vi "BT Example 6 - Parallel.vi"() -> ()   [LabVIEW 2021]
uses:
  Support/Nodes/abs_Node/Status.ctl
  Blackboard/Blackboard.lvclass
  Support/Nodes/Decorators/Repeater/Support/Finish On - Type.ctl
  Support/Nodes/Composites/abs_Parallel/Support/Status Calculation.ctl
  System/bt_System.lvclass
  Blackboard/Blackboard.lvclass/Blackboard.ctl
  Support/Nodes/Leaves/abs_Type Leaf/abs_Type Leaf.lvclass/abs_Type Leaf.ctl
  Blackboard/Get Value Type/Get I32.vi
  <vilib>/TSA/Abstract Data Classes/Abs_Types/I32 Integer/Static Read.vi
  Blackboard/Support/Index Group.vi
  Blackboard/Support/Index Tags.vi
  Support/Nodes/Leaves/abs_Type Leaf/Properties/Write Value Class.vi
  <vilib>/TSA/Omni-Bus/Local Bus/Support/I32/Local Bus_I32.lvclass
  C:/Program Files (x86)/National Instruments/LabVIEW 2021/vi.lib/TSA/Abstract Data Classes/Abs_Types/Value/Abs_Value.lvclass
  <vilib>/TSA/Abstract Data Classes/Abs_Types/I32 Integer/Abs_I32 Integer.lvclass
  Support/Nodes/Leaves/Test Boolean/Test Abs_Boolean.lvclass
  C:/Users/Tim/Documents/GitHub/LV_Behaviour_Tree/Source/Support/Nodes/abs_Node/bt_Node.lvclass
  C:/Users/Tim/Documents/GitHub/LV_Behaviour_Tree/Source/Support/Nodes/Leaves/abs_Type Leaf/abs_Type Leaf.lvclass
  <vilib>/TSA/Abstract Data Classes/Abs_Types/Boolean/Abs_Boolean.lvclass
  C:/Program Files (x86)/National Instruments/LabVIEW 2021/vi.lib/TSA/Abstract Data Classes/Abs_Types/Type/Abs_Type.lvclass
  <vilib>/TSA/Omni-Bus/Local Bus/Support/Initialise DVR's.vi
  <vilib>/TSA/Abstract Data Classes/Functions/Math/Support/Increment/I32/Method.vi
  <vilib>/TSA/Abstract Data Classes/Constants/Support/I32/I32.vi
  <vilib>/TSA/Abstract Data Classes/Functions/Math/Support/Add/I32/Method_Const.vi
  <vilib>/TSA/Abstract Data Classes/Functions/Compare/Support/Less/I32/Method_Const.vi
  <vilib>/TSA/Abstract Data Classes/Abs_Types/Value/Abs_Value.lvclass
  <vilib>/TSA/Abstract Data Classes/Abs_Types/Type/Abs_Type.lvclass
  <vilib>/TSA/Omni-Bus/Local Bus/Support/DBL/Local Bus_DBL.lvclass
  <vilib>/TSA/Omni-Bus/Local Bus/Support/SGL/Local Bus_SGL.lvclass
  <vilib>/TSA/Omni-Bus/Local Bus/Support/EXT/Local Bus_EXT.lvclass
  <vilib>/TSA/Omni-Bus/Local Bus/Support/Bool/Local Bus_Boolean.lvclass
  <vilib>/TSA/Omni-Bus/Local Bus/Support/STR/Local Bus_String.lvclass
  <vilib>/TSA/Omni-Bus/Local Bus/Support/Variant/Local Bus_Variant.lvclass
  <vilib>/TSA/Omni-Bus/Local Bus/Support/WFM/Local Bus_Waveform.lvclass
  <vilib>/TSA/Omni-Bus/Local Bus/Support/Time/Local Bus_Time.lvclass
  <vilib>/TSA/Omni-Bus/Local Bus/Support/U8/Local Bus_U8.lvclass
  <vilib>/TSA/Omni-Bus/Local Bus/Support/U16/Local Bus_U16.lvclass
  <vilib>/TSA/Omni-Bus/Local Bus/Support/U32/Local Bus_U32.lvclass
  <vilib>/TSA/Omni-Bus/Local Bus/Support/U64/Local Bus_U64.lvclass
  <vilib>/TSA/Omni-Bus/Local Bus/Support/I8/Local Bus_I8.lvclass
  <vilib>/TSA/Omni-Bus/Local Bus/Support/I16/Local Bus_I16.lvclass
  <vilib>/TSA/Omni-Bus/Local Bus/Support/I64/Local Bus_I64.lvclass
  <vilib>/TSA/Omni-Bus/Local Bus/Support/CSGL/Local Bus_CSGL.lvclass
  <vilib>/TSA/Omni-Bus/Local Bus/Support/CDBL/Local Bus_CDBL.lvclass
  <vilib>/TSA/Omni-Bus/Local Bus/Support/CEXT/Local Bus_CEXT.lvclass
  BT.lvlib
  Support/Nodes/Decorators/Repeater/bt_Repeater.lvclass
  Support/Nodes/Composites/abs_Parallel/bt_Parallel.lvclass
  <vilib>/TSA/Abstract Data Classes/Functions/Math/Support/Increment/I32/Increment_I32.lvclass
  <vilib>/TSA/Abstract Data Classes/Functions/Compare/Support/Less/I32/Less_I32.lvclass
  Support/Nodes/abs_Node/bt_Node.lvclass
  <vilib>/TSA/Abstract Data Classes/Constants/Support/I32/Const_I32.lvclass
  <vilib>/TSA/Abstract Data Classes/Functions/Math/Support/Add/I32/Add_I32.lvclass
panel:
  out "Status":T1
  out "Counts":i32[](array[numeric])
  in  "stop":bool
  # "Count 1"
  # "Count 2"
  # "Finish Count"
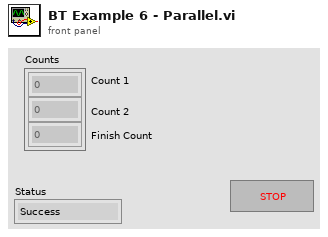
[diagram p1: front panel]
types:
  T1 = typedef "BT.lvlib/bt_Node.lvclass/Status.ctl" = enum16{"Success", "Failure", "Running"}
  T2 = typedef "BT.lvlib/bt_Parallel.lvclass/Status Calculation.ctl" = enum16{"Succeed on All Succeed", "Failure on All Failure", "Succeed on Any Succeed", "Failure on Any Failure"}
  T3 = typedef "BT.lvlib/bt_Repeater.lvclass/Finish On - Type.ctl" = enum16{"Success", "Failure", "Never"}
  T4 = typedef "Add_I32.lvclass/Abs_Type.ctl" = refnum<class "Abs_I32 Integer.lvclass">
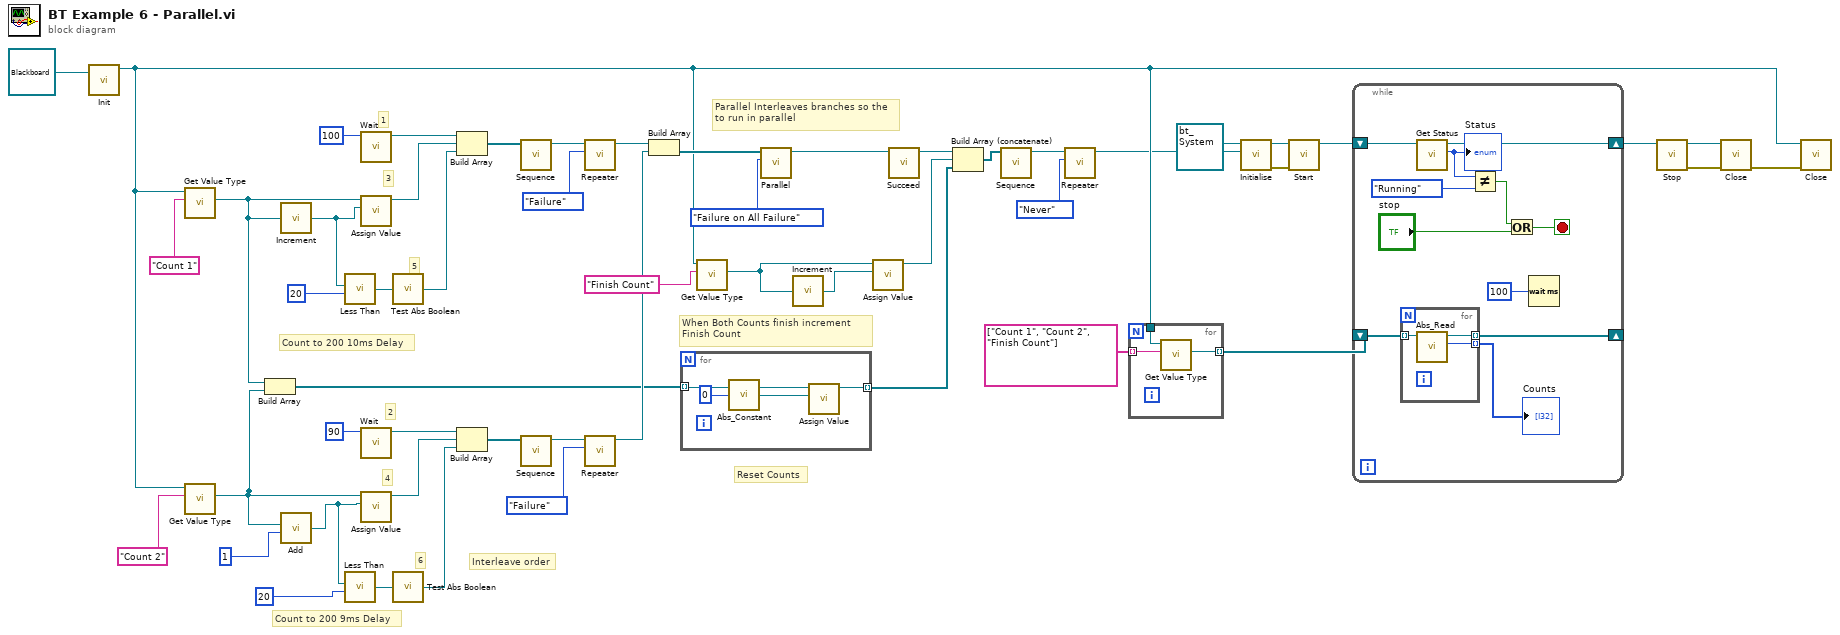
[diagram p0: block diagram]
diagram:
  # "Interleave order"
  # "6"
  # "5"
  # "4"
  # "3"
  # "2"
  # "1"
  # "Count to 200 9ms Delay"
  # "Parallel Interleaves branches so the\nto run in parallel"
  # "Reset Counts"
  # "When Both Counts finish increment\nFinish Count"
  # "Count to 200 10ms Delay"
  n1 = call-dynamic "Init.vi"("bt_Blackboard in"=refnum<class "Blackboard.lvclass"> refnum) -> ("bt_Blackboard out"=w20:refnum<class "Blackboard.lvclass">)  [unwired: 9 in, 1 out]
  n2 = call-poly "Get Value Type.vi"("Tag"="Count 1", "Blackboard in"=w20) -> ("Value"=w13:refnum<class "Abs_I32 Integer.lvclass">)  [unwired: 6 in, 3 out]
  n3 = call-poly "Get Value Type.vi"("Tag"="Count 2", "Blackboard in"=w20) -> ("Value"=w12:refnum<class "Abs_I32 Integer.lvclass">)  [unwired: 6 in, 3 out]
  n4 = Build Array(w13, w12) -> (w11:refnum<class "Abs_I32 Integer.lvclass">[])
  n5 = call-poly <vilib>:"Increment.vi"("Value"=w13) -> ("Result"=w28:refnum<class "Abs_I32 Integer.lvclass">)  [unwired: 4 in]
  n6 = call-poly <vilib>:"Add.vi"("Value"=1, "Input A"=w12) -> ("Result"=w31:T4)  [unwired: 4 in]
  n7 = call-poly <vilib>:"Less Than.vi"("Value"=20, "Value A"=w28) -> ("Result"=w29:refnum<class "Abs_Boolean.lvclass">)  [unwired: 4 in]
  n8 = call-poly <vilib>:"Less Than.vi"("Value"=20, "Value A"=w31) -> ("Result"=w30:refnum<class "Abs_Boolean.lvclass">)  [unwired: 4 in]
  n9 = call "Wait.vi"("Time (ms)"=u32 100) -> ("Node Out"=w51:refnum<class "bt_Node.lvclass">)  [unwired: 10 in]
  n10 = call "Assign Value.vi"("Assigned Value"=w28, "Value"=w13) -> ("Node Out"=w45:refnum<class "bt_Node.lvclass">)  [unwired: 9 in]
  n11 = call "Wait.vi"("Time (ms)"=u32 90) -> ("Node Out"=w38:refnum<class "bt_Node.lvclass">)  [unwired: 10 in]
  n12 = call "Assign Value.vi"("Assigned Value"=w31, "Value"=w12) -> ("Node Out"=w41:refnum<class "bt_Node.lvclass">)  [unwired: 9 in]
  n13 = call "Test Abs Boolean.vi"("Abs_Boolean.lvclass"=w29) -> ("abs_Node"=w14:refnum<class "bt_Node.lvclass">)  [unwired: 4 in]
  n14 = call "Test Abs Boolean.vi"("Abs_Boolean.lvclass"=w30) -> ("abs_Node"=w16:refnum<class "bt_Node.lvclass">)  [unwired: 4 in]
  n15 = Build Array(w51, w45, w14) -> (w50:refnum<class "bt_Node.lvclass">[])
  n16 = Build Array(w38, w41, w16) -> (w39:refnum<class "bt_Node.lvclass">[])
  n17 = call "Sequence.vi"("Nodes"=w50) -> ("Node"=w37:refnum<class "bt_Node.lvclass">)  [unwired: 10 in]
  n18 = call "Sequence.vi"("Nodes"=w39) -> ("Node"=w33:refnum<class "bt_Node.lvclass">)  [unwired: 10 in]
  n19 = call "Repeater.vi"("Finish On"=Finish_On_-_Type."Failure", "Node In"=w37) -> ("Node Out"=w36:refnum<class "bt_Node.lvclass">)  [unwired: 9 in]
  n20 = call "Repeater.vi"("Finish On"=Finish_On_-_Type."Failure", "Node In"=w33) -> ("Node Out"=w32:refnum<class "bt_Node.lvclass">)  [unwired: 9 in]
  n21 = Build Array(w36, w32) -> (w27:refnum<class "bt_Node.lvclass">[])
  n22 = for {
    tunnel: [w55] -> w15 mode=indexing
    tunnel: w11 -> [w54] mode=indexing
    n23 = call-poly <vilib>:"Abs_Constant.vi"("Value"=0) -> ("Constant"=w56:refnum<class "Abs_I32 Integer.lvclass">)  [unwired: 4 in]
    n24 = call "Assign Value.vi"("Assigned Value"=w56, "Value"=w54) -> ("Node Out"=w55:refnum<class "bt_Node.lvclass">)  [unwired: 9 in]
  }
  n25 = call-poly "Get Value Type.vi"("Tag"="Finish Count", "Blackboard in"=w20) -> ("Value"=w25:refnum<class "Abs_I32 Integer.lvclass">)  [unwired: 6 in, 3 out]
  n26 = call "Parallel.vi"("Status Calculation"=Status_Calculation."Failure on All Failure", "Nodes"=w27) -> ("Node"=w19:refnum<class "bt_Node.lvclass">)  [unwired: 9 in]
  n27 = call-poly <vilib>:"Increment.vi"("Value"=w25) -> ("Result"=w24:refnum<class "Abs_I32 Integer.lvclass">)  [unwired: 4 in]
  n28 = call "Assign Value.vi"("Assigned Value"=w24, "Value"=w25) -> ("Node Out"=w17:refnum<class "bt_Node.lvclass">)  [unwired: 9 in]
  n29 = call "Succeed.vi"("Node In"=w19) -> ("Node"=w18:refnum<class "bt_Node.lvclass">)  [unwired: 10 in]
  n30 = Build Array (concatenate)(w18, w17, w15) -> (w22:refnum<class "bt_Node.lvclass">[])
  n31 = call "Sequence.vi"("Nodes"=w22) -> ("Node"=w21:refnum<class "bt_Node.lvclass">)  [unwired: 10 in]
  n32 = call "Repeater.vi"("Finish On"=Finish_On_-_Type."Never", "Node In"=w21) -> ("Node Out"=w2:refnum<class "bt_Node.lvclass">)  [unwired: 9 in]
  n33 = for {
    tunnel: string[] ["Count 1", "Count 2", "Finish Count"] ("Tag") -> [w60] mode=indexing
    tunnel: [w59] -> w43 mode=indexing
    tunnel: w20 -> [w58]
    n34 = call-poly "Get Value Type.vi"("Tag"=w60, "Blackboard in"=w58) -> ("Value"=w59:refnum<class "Abs_I32 Integer.lvclass">)  [unwired: 6 in, 3 out]
  }
  n35 = call "Initialise.vi"("Behaviour Tree"=w2, "bt_System in"=refnum<class "bt_System.lvclass"> refnum) -> ("error out"=w3:errorcluster, "bt_System out"=w4:refnum<class "bt_System.lvclass">)  [unwired: 8 in]
  n36 = call "Start.vi"("error in (no error)"=w3, "bt_System in"=w4) -> ("bt_System out"=w53:refnum<class "bt_System.lvclass">)  [unwired: 8 in, 1 out]
  n37 = while {
    shift-right: [w66] -> w52
    shift-left: w53 -> [w67]
    shift-right: [w70] -> _
    shift-left: w43 -> [w71]
    stop <- w63 stop-if-true
    n38 = for {
      tunnel: w71 -> [w74] mode=indexing
      tunnel: [w73] -> w70 mode=indexing
      tunnel: [w72] -> w69 mode=indexing
      n39 = call-poly <vilib>:"Abs_Read.vi"("Abs_I32 Integer in"=w74) -> ("Value"=w72:i32, "Abs_I32 Integer out"=w73:refnum<class "Abs_I32 Integer.lvclass">)  [unwired: 8 in, 1 out]
    }
    "Counts" <- w69
    n40 = call "Get Status.vi"("bt_System in"=w67) -> ("Status"=w65:T1, "bt_System out"=w66:refnum<class "bt_System.lvclass">)  [unwired: 8 in, 1 out]
    "Status" <- w65
    n41 = Not Equal?(x=w65, y=Status."Running") -> (x != y?=w62:bool)
    n42 = Or(x=w62, y="stop") -> (x .or. y?=w63:bool)
    n43 = Wait (ms)(milliseconds to wait=u32 100) -> ()  [unwired: 1 out]
  }
  n44 = call "Stop.vi"("bt_System in"=w52) -> ("error out"=w9:errorcluster, "bt_System out"=w10:refnum<class "bt_System.lvclass">)  [unwired: 9 in]
  n45 = call-dynamic "Close.vi"("error in (no error)"=w9, "bt_System in"=w10) -> ("error out"=w48:errorcluster)  [unwired: 8 in, 1 out]
  n46 = call-dynamic "Close.vi"("error in (no error)"=w48, "bt_Blackboard in"=w20) -> ()  [unwired: 8 in, 2 out]
